vi "Coord window-Add to picture-Coord list.vi"(7 "Feature to draw":enum16{"Draw point", "Draw square"}(ring), 10 "ItemNames":string[][](array[string]), 11 "Picture in":refnum<vi>) -> (2 "new picture":picture, 3 "Picture out":refnum<vi>)   [LabVIEW 2017]
panel:
  in  "color":u32(colorbox)=28055
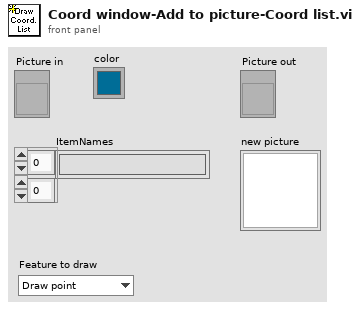
[diagram p1: front panel]
types:
  T1 = cluster{"left":i16, "top":i16, "right":i16, "bottom":i16}
  T2 = typedef "LVBoundsTypeDef.ctl" = cluster{"Width":u32, "Height":u32}
  T3 = cluster{"FOV/2-X (pixels)":i16, "FOV/2-Y (pixels)":i16}
  T4 = cluster{"Width":u16, "Style":enum32{"Solid", "Dash", "Dot", "DashDot", "DashDotDot"}}
  T5 = cluster{"Width":i16, "Style":enum32{"Solid", "Dash", "Dot", "DashDot", "DashDotDot"}}
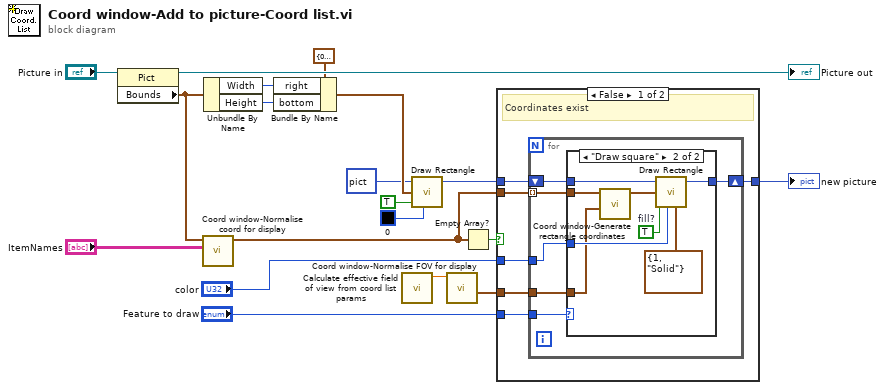
[diagram p0: block diagram]
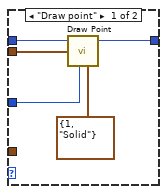
[diagram p2: hidden frame]
diagram:
  n1 = property on="Property Node" class="Pict"(reference="Picture in") -> (reference out=→"Picture out":refnum<vi>, "Bounds"=w17:T2)  [unwired: 1 in, 1 out]
  n2 = call "Coord window-Normalise coord for display.vi"("MCList ItemNames"="ItemNames", "Bounds"=w17) -> ("Normalised coordinates (for display)"=w6:cluster{"x":i16, "y":i16}[])  [unwired: 9 in]
  n3 = Unbundle By Name(w17) -> ("Width"=w8:u32, "Height"=w9:u32)
  n4 = Bundle By Name(cluster=T1 {"left"=0, "top"=0, "right"=30, "bottom"=40} ("rect"), "right"=w8, "bottom"=w9) -> (w14:T1)
  n5 = call "Calculate effective field of view from coord list params.vi"() -> ("Effective FOV (um)"=w1:sgl)  [unwired: 11 in]
  n6 = call <vilib>:"Draw Rectangle.vi"("picture"=picture data[5B] ("2D Picture"), "rect"=w14, "fill?(F)"=TRUE, "color(black)"=u32 0) -> ("new picture"=w13:picture)  [unwired: 5 in]
  n7 = call "Coord window-Normalise FOV for display.vi"("Effective FOV (um)"=w1) -> ("Normalised Effective FOV/2"=w3:T3)  [unwired: 9 in, 1 out]
  n8 = Empty Array?(array=w6) -> (empty?=w5:bool)
  n9 = case shown="False" w5 {
    tunnel: [w25 w45] -> w18
    tunnel: w6 -> [w24 _]
    tunnel: w13 -> [w23 w45]
    tunnel: "Feature to draw" -> [w22 _]
    tunnel: w3 -> [w21 _]
    tunnel: "color" -> [w20 _]
    frame False {
      # "Coordinates exist"
      n10 = for {
        shift-right: [w30] -> w25
        shift-left: w23 -> [w31]
        tunnel: w24 -> [w29] mode=indexing
        tunnel: w22 -> [w28]
        tunnel: w21 -> [w27]
        tunnel: w20 -> [w26]
        n11 = case shown="\"Draw square\"" w28 {
          tunnel: w31 -> [w36 w44]
          tunnel: [w34 w43] -> w30
          tunnel: w29 -> [w33 w41]
          tunnel: w26 -> [w32 w42]
          tunnel: w27 -> [_ w37]
          frame "Draw point" {
            n12 = call <vilib>:"Draw Point.vi"("picture"=w36, "point(x,y)"=w33, "color(black)"=w32, "pen"=T4 {"Width"=1, "Style"=enum."Solid"}) -> ("new picture"=w34:picture)  [unwired: 5 in]
          }
          frame "Draw square" {
            w38 = TRUE  # fill?
            n13 = call "Coord window-Generate rectangle coordinates.vi"("Normalised Effective FOV/2"=w37, "Norm point(x,y) (for display)"=w41) -> ("Norm rect (for display)"=w40:T1)  [unwired: 9 in]
            n14 = call <vilib>:"Draw Rectangle.vi"("picture"=w44, "rect"=w40, "fill?(F)"=w38, "color(black)"=w42, "pen"=T5 {"Width"=1, "Style"=enum."Solid"}) -> ("new picture"=w43:picture)  [unwired: 4 in]
          }
        }
      }
    }
    frame True {
      # "No coordinates exist"
    }
  }
  "new picture" <- w18
